vi "SI8_Parsing_data_num.vi"(11 "Input":string) -> (3 "Choice":string)   [LabVIEW 2018]
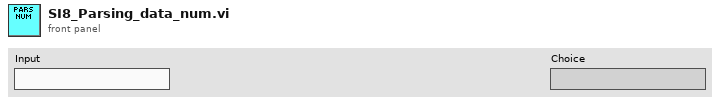
[diagram p1: front panel]
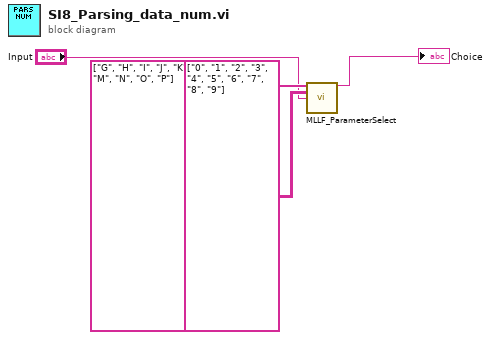
[diagram p0: block diagram]
diagram:
  n1 = call "MLLF_ParameterSelect.vi"("Command to equipment"=string[] ["0", "1", "2", "3", "4", "5", "6", "7", "8", "9"] ("Command 2 equipment"), "Names"=string[][] [["G"], ["H"], ["I"], ["J"], ["K"], ["L"], ["M"], ["N"], ["O"], ["P"]], "Input"="Input") -> ("Choice"=→"Choice":string)  [unwired: 11 in, 1 out]
